vi "Start Sync.vi"(8 "error in (no error)":errorcluster, 11 "gRPC Server in":refnum<class "GreeterService.lvclass">) -> (0 "error out":errorcluster, 3 "gRPC Server out":refnum<class "GreeterService.lvclass">)   [LabVIEW 2019, in "Generated_server.lvlib" / "GreeterService.lvclass"]
uses:
  GreeterService.lvclass
  RPC Messages/Greeter_req_req_oneof/Greeter_req_req_oneof.lvclass
  RPC Messages/Greeter_res_res_oneof/Greeter_res_res_oneof.lvclass
  RPC Messages/Greeter_res.ctl
  Generated_server.lvlib
  RPC Messages/Greeter_MessageA.ctl
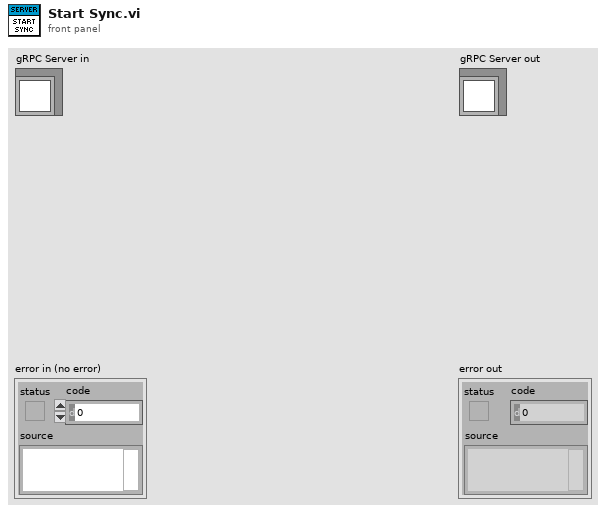
[diagram p1: front panel]
types:
  T1 = typedef "Generated_server.lvlib/Greeter_res.ctl" = cluster{"res_latitude":i32, "Greeter_res_res_oneof":refnum<class "Greeter_res_res_oneof.lvclass">, "message_a":T2}
  T2 = typedef "Generated_server.lvlib/Greeter_MessageA.ctl" = cluster{"data_a1":string}
  T3 = typedef "Generated_server.lvlib/GreeterService.lvclass/Server Internal UEs.ctl" = cluster{"GreeterService GetFeature Internal UE":refnum<user-event>}
  T4 = typedef "Generated_server.lvlib/GreeterService.lvclass/Server gRPC UEs.ctl" = cluster{"GreeterService GetFeature gRPC UE":refnum<user-event>}
  T5 = typedef "grpc-lvsupport-release.lvlib/grpcId.ctl" = u64
  T6 = typedef "Generated_server.lvlib/Greeter_req.ctl" = cluster{"req_latitude":i32, "message_a":T2, "Greeter_req_req_oneof":refnum<class "Greeter_req_req_oneof.lvclass">}
  T7 = typedef "grpc-lvsupport.lvlib/grpcId.ctl" = u64
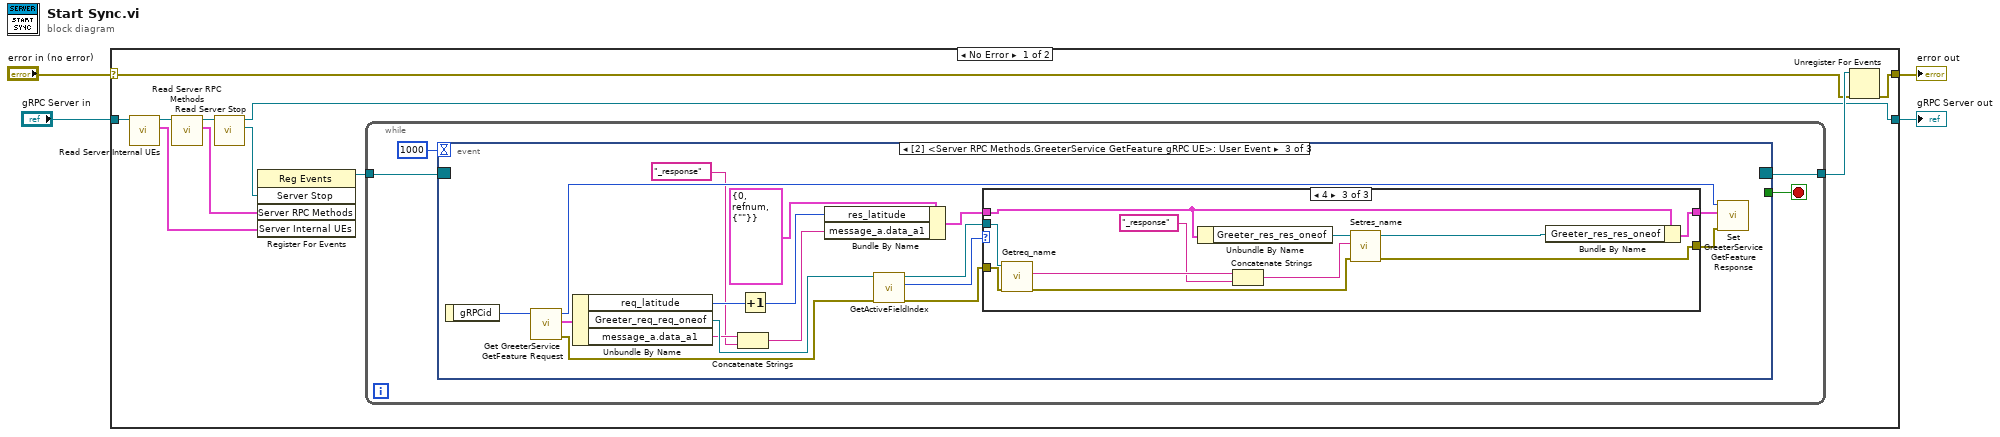
[diagram p0: block diagram]
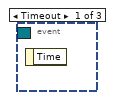
[diagram p2: hidden frame]
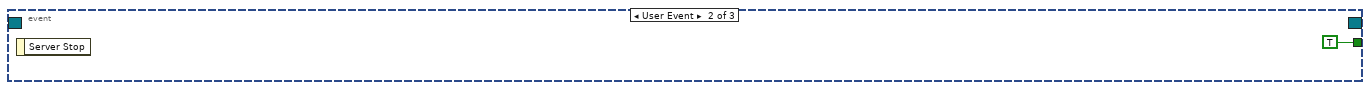
[diagram p3: hidden frame]
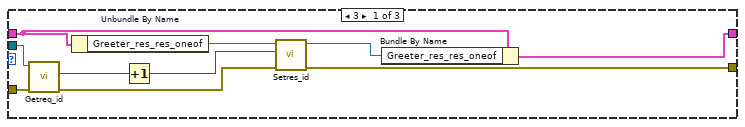
[diagram p4: hidden frame]
diagram:
  n1 = case shown="No Error" "error in (no error)" {
    selector: "error in (no error)" -> [w9 w62]
    tunnel: [w8 w62] -> w3
    tunnel: [w6 w61] -> w1
    tunnel: "gRPC Server in" -> [w15 w61]
    frame No Error {
      n2 = call "Read Server Internal UEs.vi"("SignalGeneratorService in"=w15) -> ("Server Internal UEs"=w13:T3, "SignalGeneratorService out"=w14:refnum<class "GreeterService.lvclass">)  [unwired: 8 in, 1 out]
      n3 = call "Read Server RPC Methods.vi"("SignalGeneratorService in"=w14) -> ("Server RPC Methods"=w7:T4, "SignalGeneratorService out"=w12:refnum<class "GreeterService.lvclass">)  [unwired: 8 in, 1 out]
      n4 = call-dynamic "Read Server Stop.vi"("iService in"=w12) -> ("Server Stop"=w5:refnum<user-event>, "iService out"=w6:refnum<class "GreeterService.lvclass">)  [unwired: 8 in, 1 out]
      n5 = register-events(w5, w7, w13) -> (reference out=w11:refnum<event-registration>)  [unwired: 2 in, 1 out]
      n6 = while {
        tunnel: w11 -> [w19]
        tunnel: [w17] -> w10
        stop <- w18 stop-if-true
        n7 = event "RPC Methods Event Structure" shown="[2] <Server RPC Methods.GreeterService GetFeature gRPC UE>: User Event" {
          selector: w19 -> [_ _ _]
          dyn-events: [_ _ _] -> w17
          timeout: 1000 -> [_ _ _]
          tunnel: [_ TRUE _] -> w18
          event Timeout {
            n8 = event-data() -> ()  [unwired: 1 in, 1 out]
          }
          event User Event {
            n9 = event-data() -> ()  [unwired: 1 in, 1 out]
          }
          event User Event {
            n10 = event-data() -> ("gRPCid"=w37:T5)  [unwired: 1 in]
            n11 = call "Get GreeterService GetFeature Request.vi"("gRPCid in"=w37) -> ("error out"=w24:errorcluster, "Message Data"=w36:T6, "gRPCid out"=w31:T7)  [unwired: 8 in]
            n12 = Unbundle By Name(w36) -> ("req_latitude"=w30:i32, "Greeter_req_req_oneof"=w35:refnum<class "Greeter_req_req_oneof.lvclass">, "message_a.data_a1"=w27:string)
            n13 = Concatenate Strings(w27, "_response" ("string")) -> (w26:string)
            n14 = Increment(x=w30) -> (x+1=w29:i32)
            n15 = Bundle By Name(cluster=T1 {"res_latitude"=0, "Greeter_res_res_oneof"=refnum, "message_a"={"data_a1"=""}} ("Greeter_res"), "res_latitude"=w29, "message_a.data_a1"=w26) -> (w28:T1)
            n16 = call "GetActiveFieldIndex.vi"("error in (no error)"=w24, "OneOfTemplate in"=w35) -> ("error out"=w22:errorcluster, "Active Field Index"=w34:i32, "OneOfTemplate out"=w33:refnum<class "Greeter_req_req_oneof.lvclass">)  [unwired: 7 in]
            n17 = case shown="4" w34 {
              tunnel: w28 -> [w47 w49 w56]
              tunnel: w33 -> [w44 _ w60]
              tunnel: [w46 w49 w53] -> w23
              tunnel: w22 -> [w45 w48 w52]
              tunnel: [w38 w48 w50] -> w21
              frame 3 {
                n18 = call "Getreq_id.vi"("error in (no error)"=w45, "OneOfTemplate in"=w44) -> ("error out"=w43:errorcluster, "Get_Val"=w42:i32)  [unwired: 7 in, 1 out]
                n19 = Unbundle By Name(w47) -> ("Greeter_res_res_oneof"=w40:refnum<class "Greeter_res_res_oneof.lvclass">)
                n20 = Increment(x=w42) -> (x+1=w41:i32)
                n21 = call "Setres_id.vi"("error in (no error)"=w43, "Set_Val"=w41, "OneOfTemplate in"=w40) -> ("error out"=w38:errorcluster, "OneOfTemplate out"=w39:refnum<class "Greeter_res_res_oneof.lvclass">)  [unwired: 7 in]
                n22 = Bundle By Name(cluster=w47, "Greeter_res_res_oneof"=w39) -> (w46:T1)
              }
              frame 0, Default {
              }
              frame 4 {
                n23 = call "Getreq_name.vi"("error in (no error)"=w52, "OneOfTemplate in"=w60) -> ("error out"=w51:errorcluster, "Get_Val"=w59:string)  [unwired: 7 in, 1 out]
                n24 = Unbundle By Name(w56) -> ("Greeter_res_res_oneof"=w55:refnum<class "Greeter_res_res_oneof.lvclass">)
                n25 = Concatenate Strings(w59, "_response" ("string")) -> (w57:string)
                n26 = call "Setres_name.vi"("error in (no error)"=w51, "Set_Val"=w57, "OneOfTemplate in"=w55) -> ("error out"=w50:errorcluster, "OneOfTemplate out"=w54:refnum<class "Greeter_res_res_oneof.lvclass">)  [unwired: 7 in]
                n27 = Bundle By Name(cluster=w56, "Greeter_res_res_oneof"=w54) -> (w53:T1)
              }
            }
            n28 = call "Set GreeterService GetFeature Response.vi"("error in (no error)"=w21, "Message Data"=w23, "gRPCid in"=w31) -> ()  [unwired: 8 in, 1 out]
          }
        }
      }
      n29 = Unregister For Events(event registration refnum=w10, error in=w9) -> (error out=w8:errorcluster)
    }
    frame Error {
    }
  }
  "error out" <- w3
  "gRPC Server out" <- w1
